vi "SRVSettings.vi"(8 "error in (no error)":errorcluster, 11 "SRV IP Address":string) -> (0 "error out":errorcluster, 1 "Cancelled?":bool, 3 "SRV IP Address out":string)   [LabVIEW 2009]
doc: "Modified for Benilde St. Margaret's School - Tim Jump\nBy Doug Schmertman - Logic PD\nCopyright 2012"
panel:
  # "This LabVIEW item is deprecated.\n\nIt is believed to be unused and will be removed in a future version of SRV."
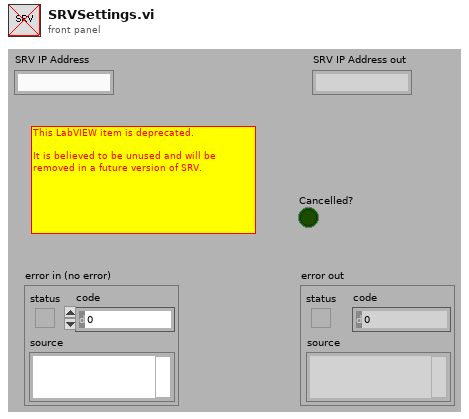
[diagram p1: front panel]
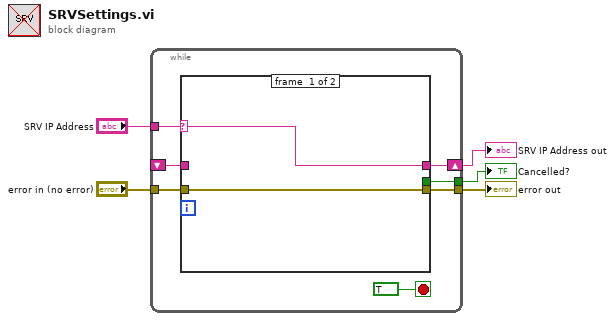
[diagram p0: block diagram]
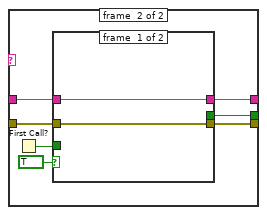
[diagram p2: hidden frame]
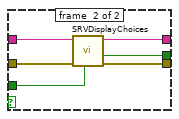
[diagram p3: hidden frame]
diagram:
  n1 = while {
    tunnel: "SRV IP Address" -> [w11]
    shift-right: [w12] -> w5
    shift-left: _ -> [w9]
    tunnel: "error in (no error)" -> [w8]
    tunnel: [w7] -> w2
    tunnel: [w6] -> w1
    stop <- TRUE stop-if-true
    n2 = case shown="\"\"" w11 {
      selector: w11 -> [w14 _]
      tunnel: [w14 w20] -> w12
      tunnel: w9 -> [_ w21]
      tunnel: w8 -> [w13 w19]
      tunnel: [w13 w18] -> w7
      tunnel: [_ w17] -> w6
      frame #0 {
      }
      frame #1 {
        n3 = First Call?() -> (First Call?: T/F=w15:bool)
        n4 = case shown="True" TRUE {
          tunnel: w21 -> [w23 w29]
          tunnel: [w23 w28] -> w20
          tunnel: w19 -> [w22 w27]
          tunnel: [w22 w26] -> w18
          tunnel: [_ w25] -> w17
          tunnel: w15 -> [_ w24]
          frame #0 {
          }
          frame #1 {
            n5 = call "SRVDisplayChoices.vi"("Delete INI File First? (F)"=w24, "error in (no error)"=w27, "SRV IP Address"=w29) -> ("error out"=w26:errorcluster, "Cancelled?"=w25:bool, "SRV IP Address out"=w28:string)  [unwired: 6 in]
          }
        }
      }
    }
  }
  "SRV IP Address out" <- w5
  "error out" <- w2
  "Cancelled?" <- w1
